vi "Write Key (Boolean).vi"(7 "Section Name":string, 8 "error in (no error)":errorcluster, 9 "Value":bool, 10 "Key Name":string, 11 "Config in":refnum<class "LabVIEW-Config.lvclass">) -> (0 "error out":errorcluster, 2 "Key Replaced?":bool, 3 "Config out":refnum<class "LabVIEW-Config.lvclass">)   [LabVIEW 2017, in "LabVIEW-Config.lvlib" / "LabVIEW-Config.lvclass"]
uses:
  LabVIEW-Config.lvclass
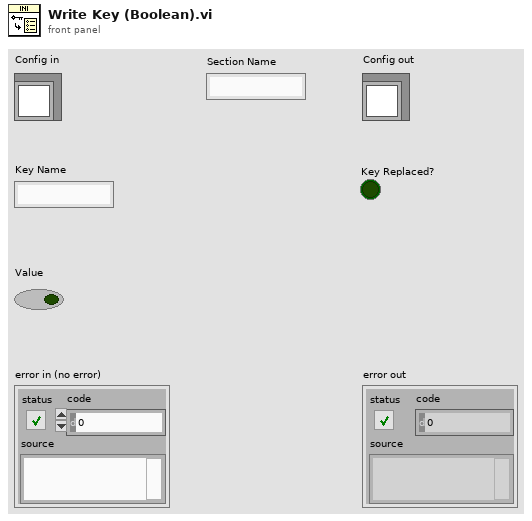
[diagram p1: front panel]
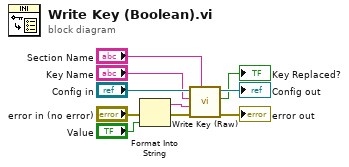
[diagram p0: block diagram]
diagram:
  n1 = Format Into String(error in="error in (no error)", "Value") -> (resulting string=w3:string, error out=w1:errorcluster)  [unwired: 2 in]
  n2 = call "Write Key (Raw).vi"("Section Name"="Section Name", "error in (no error)"=w1, "Content"=w3, "Key Name"="Key Name", "Config in"="Config in") -> ("error out"=→"error out":errorcluster, "Key Replaced?"=→"Key Replaced?":bool, "Config out"=→"Config out":refnum<class "LabVIEW-Config.lvclass">)  [unwired: 4 in]
